vi "cut_analog_input_sampling_window.vi"(9 "Sampling Frequency [Hz]":dbl=2500.0, 10 "Sampling Window [s]":dbl, 11 "elements":cluster{"Volt":dbl[]}[](array[cluster])) -> (2 "Window Size":dbl, 3 "Volt":dbl[][](array[numeric]))   [LabVIEW 2025, in "LabJackEKG.lvlib"]
uses:
  LabJackEKG.lvlib
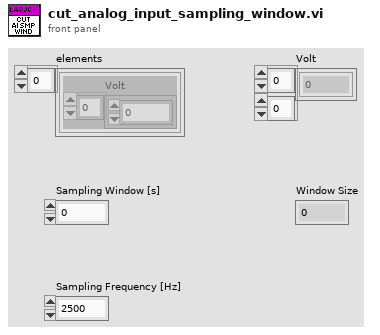
[diagram p1: front panel]
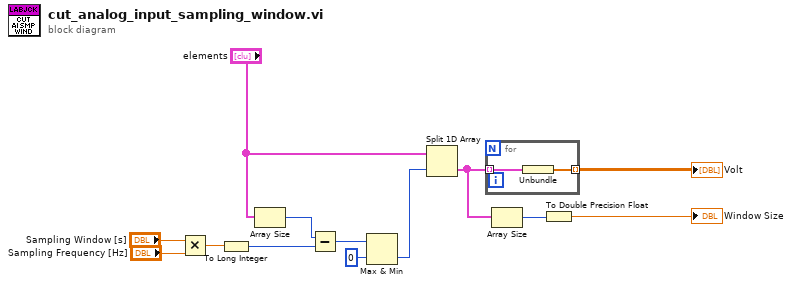
[diagram p0: block diagram]
diagram:
  n1 = Multiply(x="Sampling Window [s]", y="Sampling Frequency [Hz]") -> (x*y=w7:dbl)
  n2 = To Long Integer(number=w7) -> (32bit integer=w9:i32)
  n3 = Array Size(array="elements") -> (size(s)=w8:i32)
  n4 = Subtract(x=w8, y=w9) -> (x-y=w12:i32)
  n5 = Max & Min(x=w12, y=0) -> (min(x,y)=w11:i32)  [unwired: 1 out]
  n6 = Split 1D Array(array="elements", index=w11) -> (second subarray=w1:cluster{"Volt":dbl[]}[])  [unwired: 1 out]
  n7 = for {
    tunnel: w1 -> [w15] mode=indexing
    tunnel: [w14] -> w4 mode=indexing
    n8 = Unbundle(w15) -> ("Volt"=w14:dbl[])
  }
  "Volt" <- w4
  n9 = Array Size(array=w1) -> (size(s)=w2:i32)
  n10 = To Double Precision Float(number=w2) -> (double precision float=→"Window Size":dbl)
